vi "Puff_Dose.vi"() -> (5 "Plug in titles":string[](array[string]), 7 "Plug in values":string[](array[string]))   [LabVIEW 2012]
uses:
  Globals/Meas_global.vi
  <vilib>/Analysis/baseanly.llb/Mean (DBL).vi
  <vilib>/Analysis/NI_AALBase.lvlib
panel:
  out "D'/Dmean":dbl
  out "St Dev of Dose":dbl format="%0.2f"
  out "Mean Dose":dbl format="%0.2f"
  out "Current Block No":i32=51
  out "XY Graph":cluster{"Time (s)":dbl[], "Eng Values":dbl[]}[](graph)
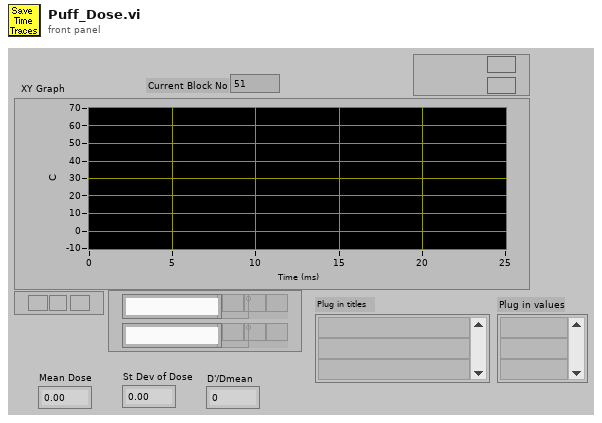
[diagram p1: front panel]
types:
  T1 = typedef "Analysis_info_cluster.ctl" = cluster{"Colour":u32, "Inst type":T2, "Inst name":string, "Symbol":string, "Code name":string, "Extra Info":string, "Inst Array":T3, "Extra Titles":string[], "Extra Values":string[], "U":dbl, "u^2":dbl, "u^3":dbl, "u^4":dbl, "Skew_u":dbl, "Kurt_u":dbl, "Sd Error in Mean":dbl, "% u'/U":dbl, "X":dbl, "Y":dbl, "Z":dbl, "Timescale integral to 25%":dbl, "Sd Error in Variance":dbl, "Calib File":path, "Calib Constants":dbl[], "Output Position":bool, "Full Stats":bool, "Av Sampling Rate":dbl, "Av No of Samples":dbl, "Total Meas Time (s)":dbl, "ADAM Ch Name":string}
  T2 = typedef "Inst_type.ctl" = enum16{"Propeller anemometer", "Raw voltage", "Pressure Transducer", "Pitot-static tube", "Preston tube", "Hot wire", "Cross wire 1", "Cross wire 2", "Generic Linear", "Generic Polynomial", "Generic BackPoly", "Fast FID", "Thermocouple", "Cold wire", "Pulsed Wire", "LDA Vel", "LDA Tran time", "LDA Arr time"}
  T3 = typedef "Instrument_Array.ctl" = enum16{"PWA", "LDA", "Analogue"}
  T4 = typedef "Time_Trace_Cluster.ctl" = cluster{"Weighting":dbl[], "Time (s)":dbl[], "Voltage":dbl[], "Eng Values":dbl[]}
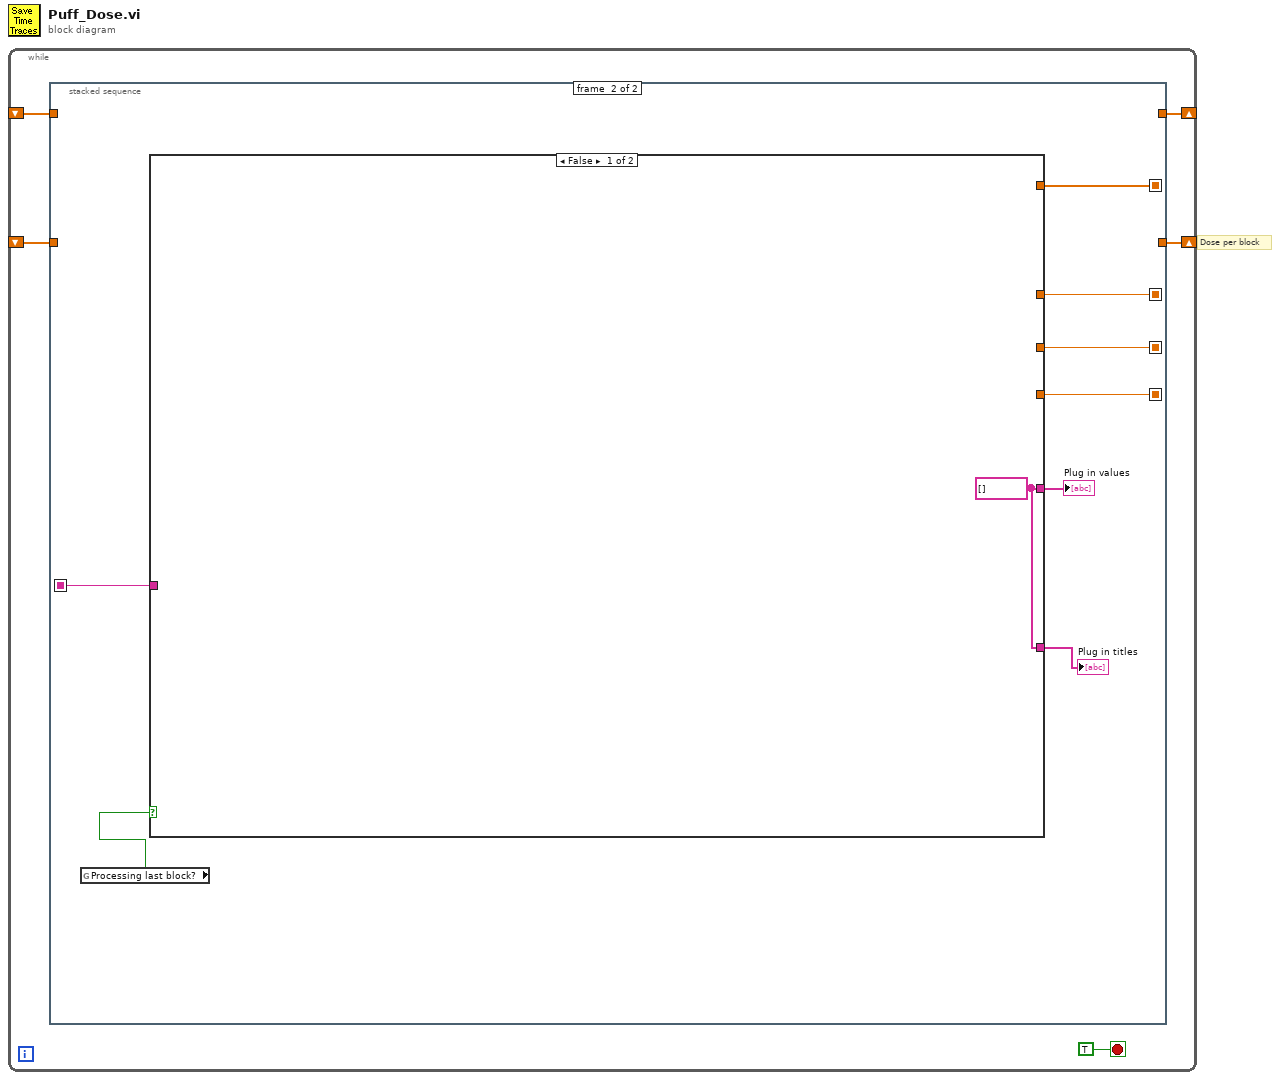
[diagram p0: block diagram]
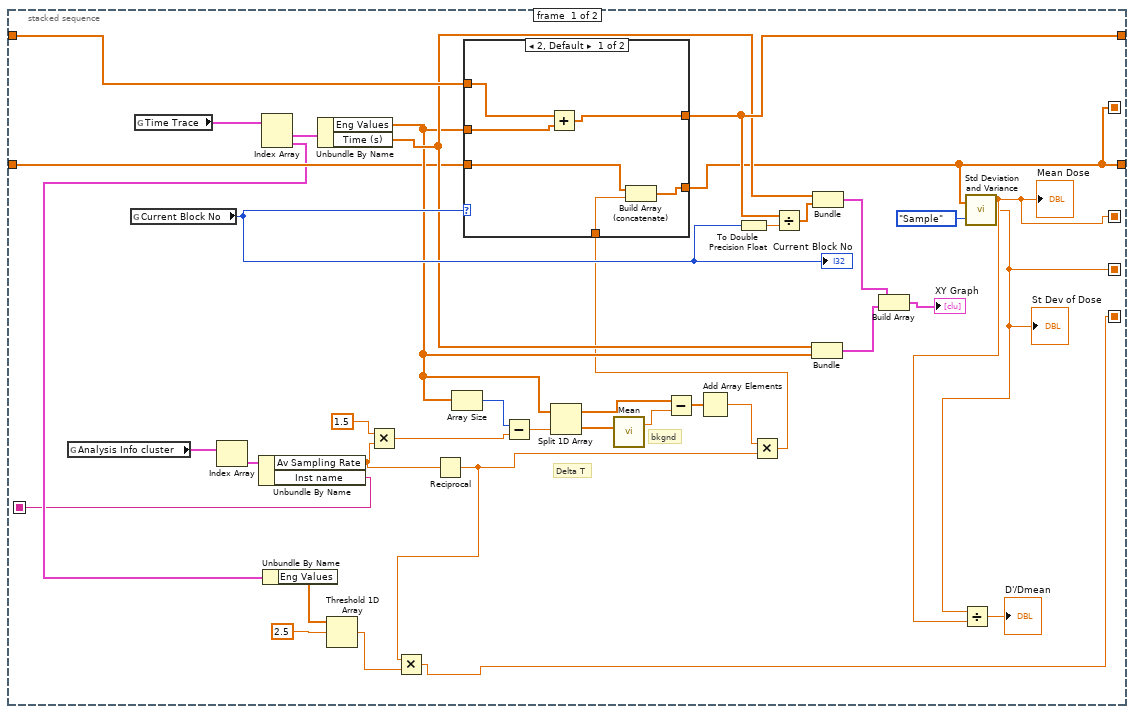
[diagram p2: hidden frame]
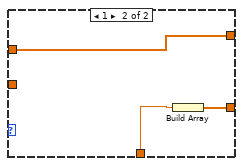
[diagram p3: hidden frame]
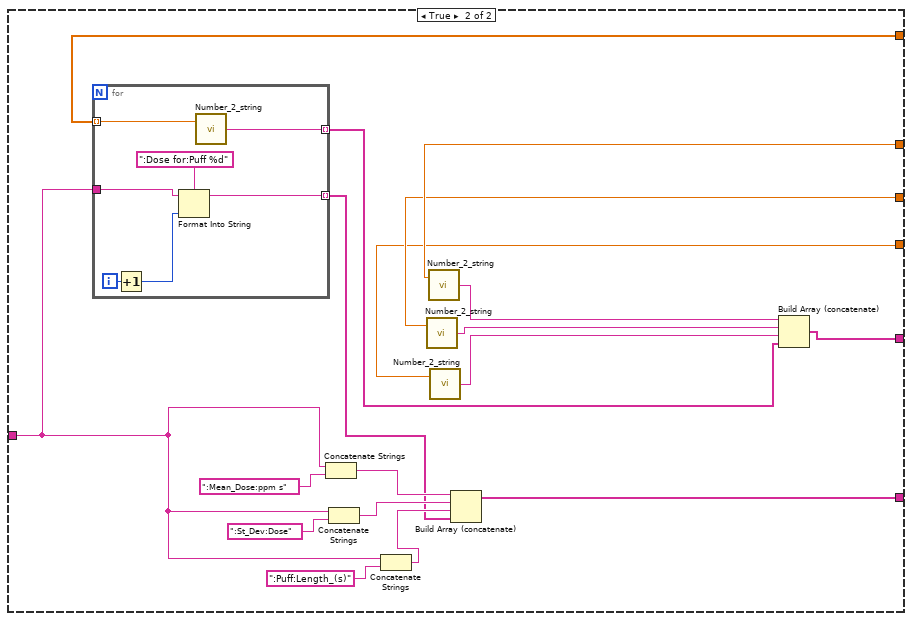
[diagram p4: hidden frame]
diagram:
  # "Dose per block"
  n1 = while {
    shift-right: [w3] -> _
    shift-left: _ -> [w5]
    shift-right: [w1] -> _
    shift-left: _ -> [w2]
    stop <- TRUE stop-if-true
    n2 = stacked-sequence {
      seq-local: [w10 _] -> [_ w59]
      seq-local: [w9 _] -> [_ w58]
      seq-local: [w8 _] -> [_ w57]
      seq-local: [w7 _] -> [_ w56]
      seq-local: [w6 _] -> [_ w55]
      tunnel: w5 -> [w42 _]
      tunnel: [w39 _] -> w3
      tunnel: w2 -> [w18 _]
      tunnel: [w6 _] -> w1
      frame #0 {
        # "bkgnd"
        # "Delta T"
        n3 = global read "Meas_global.vi" "Analysis Info cluster"() -> (w32:T1[])
        n4 = global read "Meas_global.vi" "Current Block No"() -> (w40:i32)
        "Current Block No" <- w40
        n5 = global read "Meas_global.vi" "Time Trace"() -> (w43:T4[])
        n6 = Index Array(array=w32) -> (element=w31:T1)  [unwired: 1 in]
        n7 = Unbundle By Name(w31) -> ("Av Sampling Rate"=w22:dbl, "Inst name"=w7:string)
        n8 = Index Array(array=w43) -> (element #1=w37:T4, element #2=w15:T4)  [unwired: 2 in]
        n9 = Unbundle By Name(w15) -> ("Eng Values"=w14:dbl[])
        n10 = Unbundle By Name(w37) -> ("Eng Values"=w26:dbl[], "Time (s)"=w36:dbl[])
        n11 = Threshold 1D Array(2:2.5 ("threshold y"), 3:w14) -> (0:w11:dbl)  [unwired: 1 in]
        n12 = Multiply(x=1.5, y=w22) -> (x*y=w28:dbl)
        n13 = Reciprocal(x=w22) -> (1/x=w12:dbl)
        n14 = Multiply(x=w12, y=w11) -> (x*y=w8:dbl)
        n15 = Array Size(array=w26) -> (size(s)=w29:i32)
        n16 = Subtract(x=w29, y=w28) -> (x-y=w27:dbl)
        n17 = Split 1D Array(array=w26, index=w27) -> (first subarray=w23:dbl[], second subarray=w25:dbl[])
        n18 = call-poly <vilib>:"Mean.vi"("X"=w25) -> ("mean"=w24:dbl)  [unwired: 1 out]
        n19 = Subtract(x=w23, y=w24) -> (x-y=w21:dbl[])
        n20 = Add Array Elements(numeric array=w21) -> (sum=w20:dbl)
        n21 = To Double Precision Float(number=w40) -> (double precision float=w41:dbl)
        n22 = Multiply(x=w20, y=w12) -> (x*y=w19:dbl)
        n23 = case shown="2, Default" w40 {
          tunnel: [w47 w52] -> w39
          tunnel: w26 -> [w49 w52]
          tunnel: w42 -> [w48 _]
          tunnel: w19 -> [w46 w51]
          tunnel: [w45 w50] -> w6
          tunnel: w18 -> [w44 _]
          frame 2, Default {
            n24 = Add(x=w48, y=w49) -> (x+y=w47:dbl[])
            n25 = Build Array (concatenate)(w44, w46) -> (w45:dbl[])
          }
          frame 1 {
            n26 = Build Array(w51) -> (w50:dbl[])
          }
        }
        n27 = Divide(x=w39, y=w41) -> (x/y=w38:dbl[])
        n28 = Bundle("Time (s)"=w36, "Eng Values"=w26) -> (w35:cluster{"Time (s)":dbl[], "Eng Values":dbl[]})  [unwired: 1 in]
        n29 = Bundle("Time (s)"=w36, w38) -> (w34:cluster{"Time (s)":dbl[], dbl[]})  [unwired: 1 in]
        n30 = Build Array(w34, w35) -> (→"XY Graph":cluster{"Time (s)":dbl[], "Eng Values":dbl[]}[])
        n31 = call <vilib>:"Std Deviation and Variance.vi"("X"=w6, "Weighting (Sample)"=enum16{"Sample", "Population"}."Sample") -> ("mean"=w10:dbl, "standard deviation"=w9:dbl)  [unwired: 1 out]
        "Mean Dose" <- w10
        "St Dev of Dose" <- w9
        n32 = Divide(x=w9, y=w10) -> (x/y=→"D'/Dmean":dbl)
      }
      frame #1 {
        n33 = global read "Meas_global.vi" "Processing last block?"() -> (w60:bool)
        n34 = case shown="False" w60 {
          tunnel: w59 -> [_ w77]
          tunnel: w58 -> [_ w76]
          tunnel: w57 -> [_ w75]
          tunnel: w56 -> [_ w66]
          tunnel: w55 -> [_ w67]
          tunnel: [w61 w63] -> w54
          tunnel: [w61 w62] -> w53
          frame False {
            w61 = string[] []
          }
          frame True {
            n35 = for {
              tunnel: w67 -> [w86] mode=indexing
              tunnel: w66 -> [w84]
              tunnel: [w81] -> w65 mode=indexing
              tunnel: [w80] -> w64 mode=indexing
              i -> [w85]
              n36 = Increment(x=w85) -> (x+1=w82:i32)
              n37 = Format Into String(format string=":Dose for:Puff %d", initial string=w84, w82) -> (resulting string=w80:string)  [unwired: 1 in, 1 out]
              n38 = call "Number_2_string.vi"("number"=w86) -> ("String"=w81:string)  [unwired: 1 in]
            }
            n39 = Concatenate Strings(w66, ":Mean_Dose:ppm s" ("string")) -> (w70:string)
            n40 = Concatenate Strings(w66, ":St_Dev:Dose" ("string")) -> (w69:string)
            n41 = Concatenate Strings(w66, ":Puff:Length_(s)" ("string")) -> (w68:string)
            n42 = call "Number_2_string.vi"("number"=w76) -> ("String"=w79:string)  [unwired: 1 in]
            n43 = call "Number_2_string.vi"("number"=w77) -> ("String"=w78:string)  [unwired: 1 in]
            n44 = call "Number_2_string.vi"("number"=w75) -> ("String"=w74:string)  [unwired: 1 in]
            n45 = Build Array (concatenate)(w70, w69, w68, w64) -> (w62:string[])
            n46 = Build Array (concatenate)(w78, w79, w74, w65) -> (w63:string[])
          }
        }
        "Plug in titles" <- w53
        "Plug in values" <- w54
      }
    }
  }
